vi "CRYSave Recnet.vi"   [LabVIEW 2013]
doc: "Config File Reading/Writting\n\nPath \n ini File path\nRWFlag\n 0: no action\n 1: read\n 2: write"
uses:
  CRYMainGlobal.vi
panel:
  # "Save recent configuration."
types:
  T1 = cluster{"Section":string, "Item":cluster{"Key":string, "Value":string}[]}
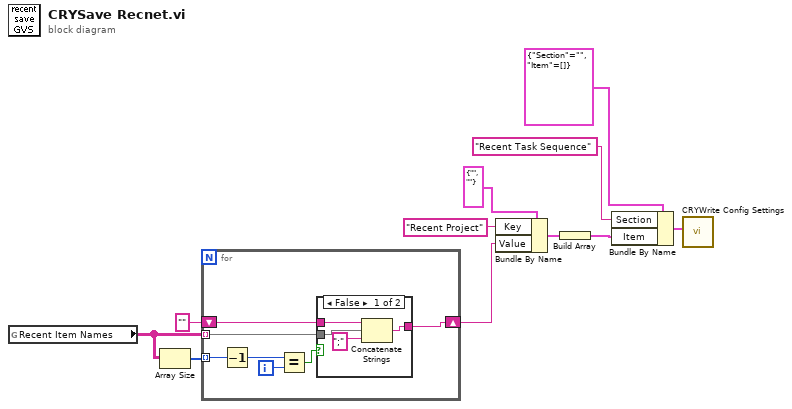
[diagram p0: block diagram]
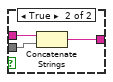
[diagram p2: hidden frame]
diagram:
  n1 = global read "CRYMainGlobal.vi" "Recent Item Names"() -> (w10:string[][])
  n2 = Array Size(array=w10) -> (size(s)=w11:i32[])
  n3 = for {
    tunnel: w10 -> [w18] mode=indexing
    shift-right: [w17] -> w4
    shift-left: "" -> [w16]
    tunnel: w11 -> [w14] mode=indexing
    i -> [w15]
    n4 = Decrement(x=w14) -> (x-1=w13:i32)
    n5 = Equal?(x=w13, y=w15) -> (x = y?=w12:bool)
    n6 = case shown="False" w12 {
      tunnel: w18 -> [w22 w24]
      tunnel: [w21 w23] -> w17
      tunnel: w16 -> [w20 w25]
      frame False {
        n7 = Concatenate Strings(w20, w22, ";" ("string")) -> (w21:string)
      }
      frame True {
        n8 = Concatenate Strings(w25, w24) -> (w23:string)
      }
    }
  }
  n9 = Bundle By Name(cluster=cluster{"Key":string, "Value":string} {"Key"="", "Value"=""} ("Cluster"), "Key"="Recent Project" ("Section"), "Value"=w4) -> (w3:cluster{"Key":string, "Value":string})
  n10 = Build Array(w3) -> (w2:cluster{"Key":string, "Value":string}[])
  n11 = Bundle By Name(cluster=T1 {"Section"="", "Item"=[]}, "Section"="Recent Task Sequence", "Item"=w2) -> (w1:T1)
  n12 = call "CRYWrite Config Settings.vi"("Config Data"=w1) -> ()  [unwired: 1 in, 8 out]
